vi "subAddItems.vi"(6 "Shallow deps?":bool, 8 "error in (no error)":errorcluster, 9 "CDependencyQueue in":refnum<class "CDependencyQueue.lvclass">, 10 "Linker.Read Info From File":T2(array[cluster]), 11 "CDependencyInspector in":refnum<class "CDependencyInspection.lvclass">) -> (0 "error out":errorcluster, 1 "CDependencyQueue out":refnum<class "CDependencyQueue.lvclass">, 3 "CDependencyInspector out":refnum<class "CDependencyInspection.lvclass">)   [LabVIEW 2020, in "DependencyInspection.lvlib" / "CDependencyInspection.lvclass"]
uses:
  CDependencyInspection.lvclass
  <vilib>/Utility/lvfile.llb/LVFileType.ctl
  CDependencyQueue/CDependencyQueue.lvclass
  CDependencyInspection.lvclass/CDependencyInspection.ctl
  CDebugInfo/CDebugInfo.lvclass
  CDependencyList/CDependencyList.lvclass
  CDependencyList/ListGenerationOptions.ctl
  <vilib>/Utility/lvfile.llb/NI_FileType.lvlib
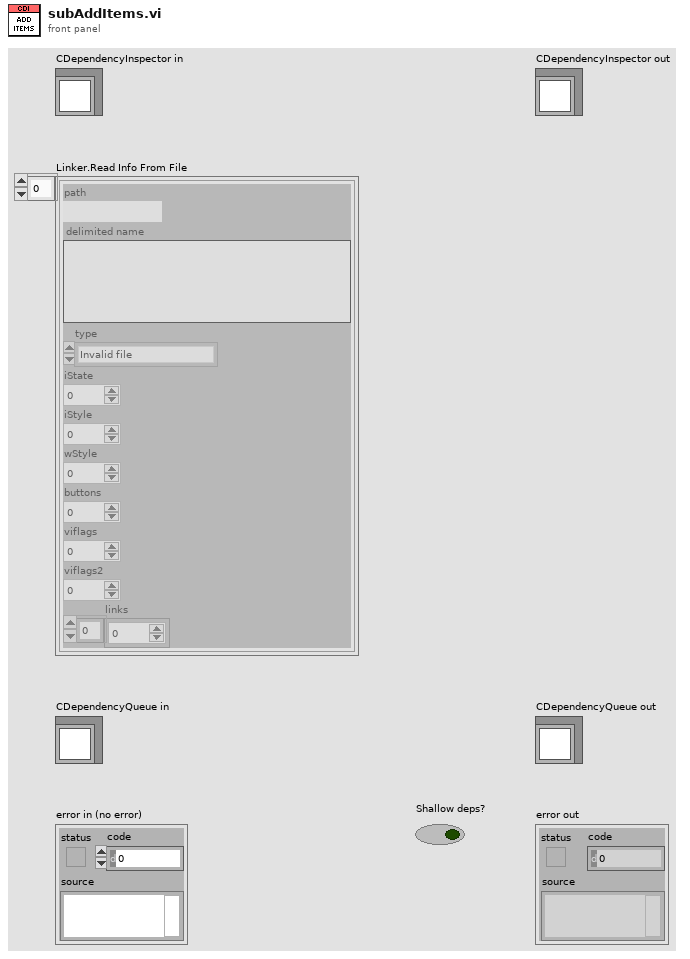
[diagram p1: front panel]
types:
  T1 = typedef "NI_FileType.lvlib/LVFileType.ctl" = enum32{"Invalid file", "Unknown type", "Instrument", "Control", "Polymorphic VI", "Project", "Library", "LVClass", "XControl", "XNode", "Shared library", ".NET assembly", "ActiveX interface", "CIN", "Run-time menu", "Palette menu", "Help file", "LLB", "XNode Edit Dependency", "Class Private Data Control", "Statechart", "MathScript .m file", "Ladder Diagram", "LVLibp", "XNode Build Dependency"}
  T2 = cluster{"path":path, "delimited name":string, "type":T1, "iState":u32, "iStyle":u16, "wStyle":u16, "buttons":u16, "viflags":u32, "viflags2":u32, "links":u32[]}[]
  T3 = typedef "DependencyInspection.lvlib/CDependencyList.lvclass/ListGenerationOptions.ctl" = cluster{"exclude external?":bool, "exclude instances?":bool, "separate tests?":bool, "Root Path":path}
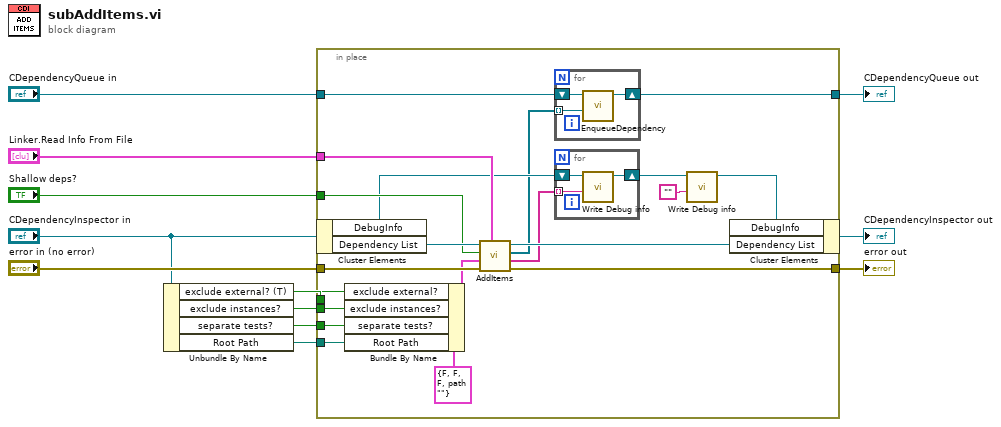
[diagram p0: block diagram]
diagram:
  n1 = Unbundle By Name("CDependencyInspector in") -> ("exclude external? (T)"=w4:bool, "exclude instances?"=w5:bool, "separate tests?"=w6:bool, "Root Path"=w9:path)
  n2 = in-place {
    in-place-border: "error in (no error)" -> [w28]
    in-place-border: "Linker.Read Info From File" -> [w29]
    in-place-border: "CDependencyQueue in" -> [w18]
    in-place-border: w9 -> [w23]
    in-place-border: [w19] -> w8
    in-place-border: [w20] -> w7
    in-place-border: w6 -> [w24]
    in-place-border: w5 -> [w25]
    in-place-border: w4 -> [w26]
    in-place-border: "Shallow deps?" -> [w27]
    n3 = in-place-cluster #1("CDependencyInspector in") -> ("DebugInfo"=w17:refnum<class "CDebugInfo.lvclass">, "Dependency List"=w30:refnum<class "CDependencyList.lvclass">)
    n4 = Bundle By Name(cluster=T3 {"exclude external?"=FALSE, "exclude instances?"=FALSE, "separate tests?"=FALSE, "Root Path"=path ""} ("Settings"), "exclude external?"=w26, "exclude instances?"=w25, "separate tests?"=w24, "Root Path"=w23) -> (w22:T3)
    n5 = call-dynamic "AddItems.vi"("Linker.Read Info From File"=w29, "error in (no error)"=w28, "Settings"=w22, "Shallow deps?"=w27, "CDependencyList in"=w30) -> ("error out"=w20:errorcluster, "Debug messages"=w15:string[], "Item to enque"=w14:refnum<class "ILabVIEWItem.lvclass">[], "CDependencyList out"=w21:refnum<class "CDependencyList.lvclass">)  [unwired: 3 in]
    n6 = for {
      shift-right: [w35] -> w19
      shift-left: w18 -> [w34]
      tunnel: w14 -> [w33] mode=indexing
      n7 = call-dynamic "EnqueueDependency.vi"("ILabVIEWItem to enqueue"=w33, "CDependencyQueue in"=w34) -> ("CDependencyQueue out"=w35:refnum<class "CDependencyQueue.lvclass">)  [unwired: 8 in, 1 out]
    }
    n8 = for {
      shift-right: [w37] -> w16
      shift-left: w17 -> [w38]
      tunnel: w15 -> [w36] mode=indexing
      n9 = call-dynamic "Write Debug info.vi"("Debug info"=w36, "CDebugInfo in"=w38) -> ("CDebugInfo out"=w37:refnum<class "CDebugInfo.lvclass">)  [unwired: 9 in]
    }
    n10 = call-dynamic "Write Debug info.vi"("Debug info"="", "CDebugInfo in"=w16) -> ("CDebugInfo out"=w32:refnum<class "CDebugInfo.lvclass">)  [unwired: 9 in]
    n11 = in-place-cluster #1("DebugInfo"=w32, "Dependency List"=w21) -> (→"CDependencyInspector out":refnum<class "CDependencyInspection.lvclass">)
  }
  "error out" <- w7
  "CDependencyQueue out" <- w8
